vi "CRYSet curve layout Front Panel.vi"(11 "Vi Ref":refnum<vi>) -> ()   [LabVIEW 2013]
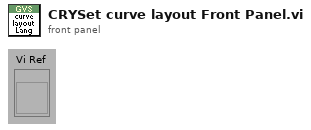
[diagram p1: front panel]
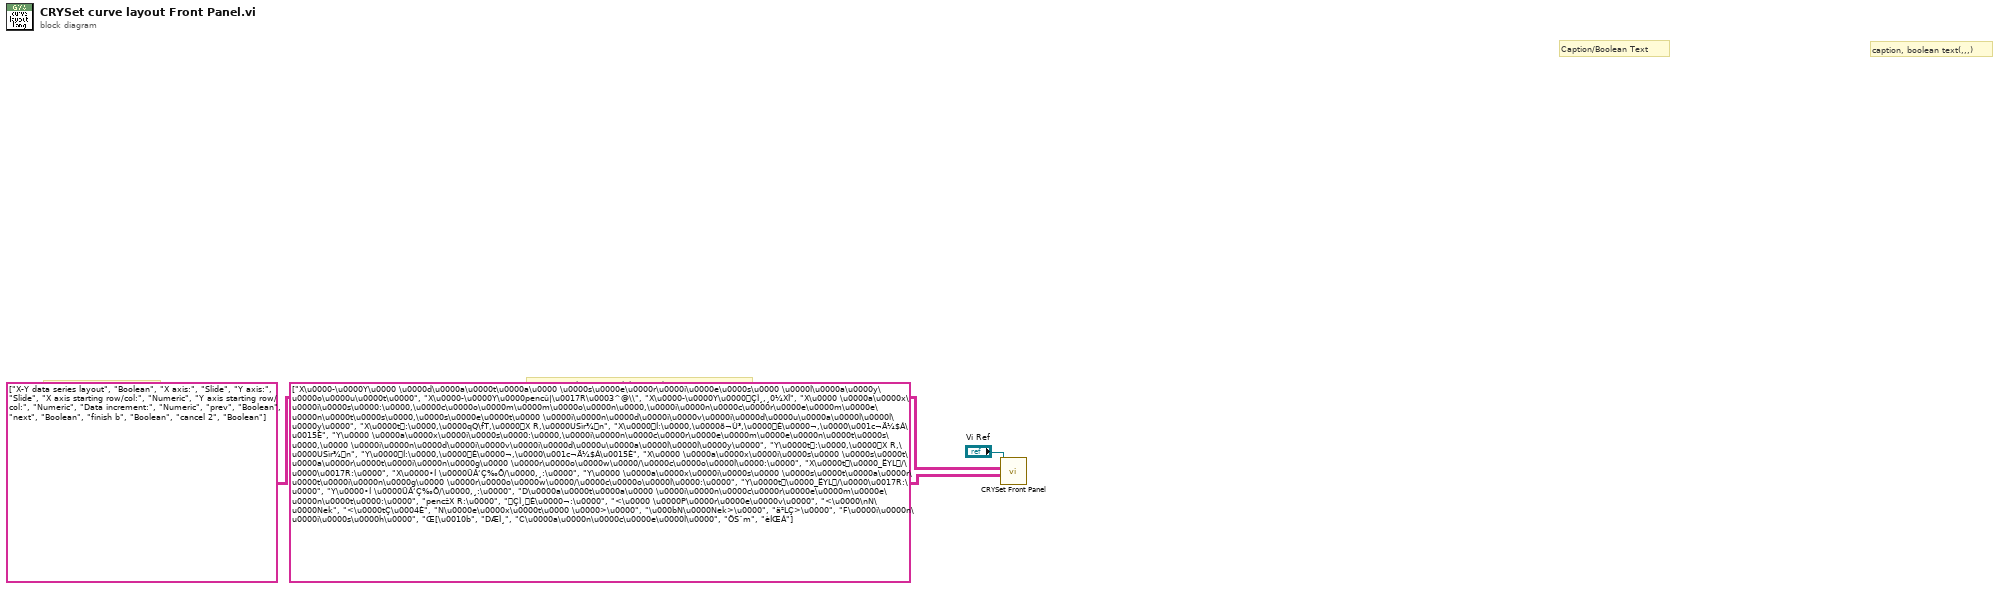
[diagram p0: block diagram]
diagram:
  # "Caption, Tab Page, Multilist Header, Button 4"
  # "Control Type"
  # "Control Name and Tab"
  # "caption, boolean text(,,,)"
  # "Caption/Boolean Text"
  n1 = call "CRYSet Front Panel.vi"("Caption(Boolean Text)"=string[][] [["X\u0000-\u0000Y\u0000 \u0000d\u0000a\u0000t\u0000a\u0000 \u0000s\u0000e\u0000r\u0000i\u0000e\u0000s\u0000 \u0000l\u0000a\u0000y\u0000o\u0000u\u0000t\u0000", "X\u0000-\u0000Y\u0000pencû|\u0017R\u0003^@\\", "X\u0000-\u0000Y\u0000ÇÌ¸,¸0¼XÎ"], ["X\u0000 \u0000a\u0000x\u0000i\u0000s\u0000:\u0000,\u0000c\u0000o\u0000m\u0000m\u0000o\u0000n\u0000,\u0000i\u0000n\u0000c\u0000r\u0000e\u0000m\u0000e\u0000n\u0000t\u0000s\u0000,\u0000s\u0000e\u0000t\u0000 \u0000i\u0000n\u0000d\u0000i\u0000v\u0000i\u0000d\u0000u\u0000a\u0000l\u0000l\u0000y\u0000", "X\u0000t:\u0000,\u0000qQ\fT,\u0000X R,\u0000USìr¾n", "X\u0000Í:\u0000,\u0000õ¬Ù³,\u0000É\u0000¬,\u0000\u001c¬Ä¼$Á\u0015È"], ["Y\u0000 \u0000a\u0000x\u0000i\u0000s\u0000:\u0000,\u0000i\u0000n\u0000c\u0000r\u0000e\u0000m\u0000e\u0000n\u0000t\u0000s\u0000,\u0000 \u0000i\u0000n\u0000d\u0000i\u0000v\u0000i\u0000d\u0000u\u0000a\u0000l\u0000l\u0000y\u0000", "Y\u0000t:\u0000,\u0000X R,\u0000USìr¾n", "Y\u0000Í:\u0000,\u0000É\u0000¬,\u0000\u001c¬Ä¼$Á\u0015È"], ["X\u0000 \u0000a\u0000x\u0000i\u0000s\u0000 \u0000s\u0000t\u0000a\u0000r\u0000t\u0000i\u0000n\u0000g\u0000 \u0000r\u0000o\u0000w\u0000/\u0000c\u0000o\u0000l\u0000:\u0000", "X\u0000t\u0000_ËYL/\u0000\u0017R:\u0000", "X\u0000•Í \u0000ÜÂ‘Ç‰Õ/\u0000,¸:\u0000"], ["Y\u0000 \u0000a\u0000x\u0000i\u0000s\u0000 \u0000s\u0000t\u0000a\u0000r\u0000t\u0000i\u0000n\u0000g\u0000 \u0000r\u0000o\u0000w\u0000/\u0000c\u0000o\u0000l\u0000:\u0000", "Y\u0000t\u0000_ËYL/\u0000\u0017R:\u0000", "Y\u0000•Í \u0000ÜÂ‘Ç‰Õ/\u0000,¸:\u0000"], ["D\u0000a\u0000t\u0000a\u0000 \u0000i\u0000n\u0000c\u0000r\u0000e\u0000m\u0000e\u0000n\u0000t\u0000:\u0000", "pencžX R:\u0000", "ÇÌ¸É\u0000¬:\u0000"], ["<\u0000 \u0000P\u0000r\u0000e\u0000v\u0000", "<\u0000\nN\u0000Nek", "<\u0000tÇ\u0004È"], ["N\u0000e\u0000x\u0000t\u0000 \u0000>\u0000", "\u000bN\u0000Nek>\u0000", "ä²LÇ>\u0000"], ["F\u0000i\u0000n\u0000i\u0000s\u0000h\u0000", "Œ[\u0010b", "DÆÌ¸"], ["C\u0000a\u0000n\u0000c\u0000e\u0000l\u0000", "ÖSˆm", "èÍŒÁ"]], "Control ID and Type(Label Name, Type)"=string[][] [["X-Y data series layout", "Boolean"], ["X axis:", "Slide"], ["Y axis:", "Slide"], ["X axis starting row/col:", "Numeric"], ["Y axis starting row/col:", "Numeric"], ["Data increment:", "Numeric"], ["prev", "Boolean"], ["next", "Boolean"], ["finish b", "Boolean"], ["cancel 2", "Boolean"]], "Vi Ref"="Vi Ref") -> ()  [unwired: 9 in]
